vi "ManageRefs_FGV.vi"(7 "ManRef_mods":T1, 8 "error in":errorcluster, 11 "DataIn":variant) -> (0 "error out":errorcluster)   [LabVIEW 2017]
uses:
  ManRef_mods.ctl
  ManRef_data.ctl
  Asteroid_data.ctl
  GameConfig/GameConfig_data.ctl
  Asteroid_states.ctl
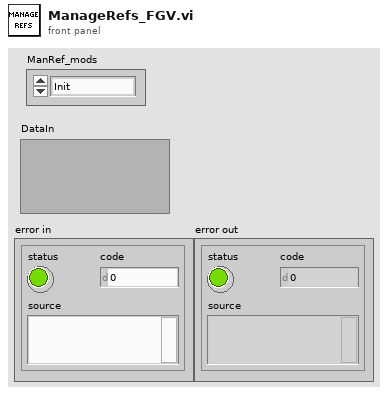
[diagram p1: front panel]
types:
  T1 = typedef "ManRef_mods.ctl" = enum16{"Init", "AddRef", "MoveAll", "DestroyRef", "End"}
  T2 = typedef "ManRef_data.ctl" = cluster{"ID":i32, "AsterObjectRef":refnum<vi>}
  T3 = typedef "Asteroid_states.ctl" = enum16{"Init", "Move", "Split", "Draw", "Destroy"}
  T4 = typedef "Asteroid_data.ctl" = cluster{"Veloc":dbl, "Direction":dbl, "Size":i32, "displayRef":refnum<vi>, "Max X":dbl, "Max Y":dbl, "Xpos":dbl, "Ypos":dbl, "ID":i32, "Config":T5}
  T5 = typedef "GameConfig_data.ctl" = cluster{"SpaceShip":cluster{"Angle":dbl, "SideLenght":dbl, "MaxLinearVeloc":dbl, "MaxAngularVeloc":dbl, "LinearAceleration":dbl, "AngularAceleration":dbl}, "Physics":cluster{"LinearDragFactor":dbl, "AngularDragFactor":dbl}, "Asteroids":cluster{"MaxSize":dbl, "MaxDivisions":i32, "MaxVeloc":dbl, "MinVeloc":dbl, "Fill":bool}, "Environment":cluster{"MaxAsteroids":i32, "TimeIncrement":dbl, "AsterProbCreation":dbl}}
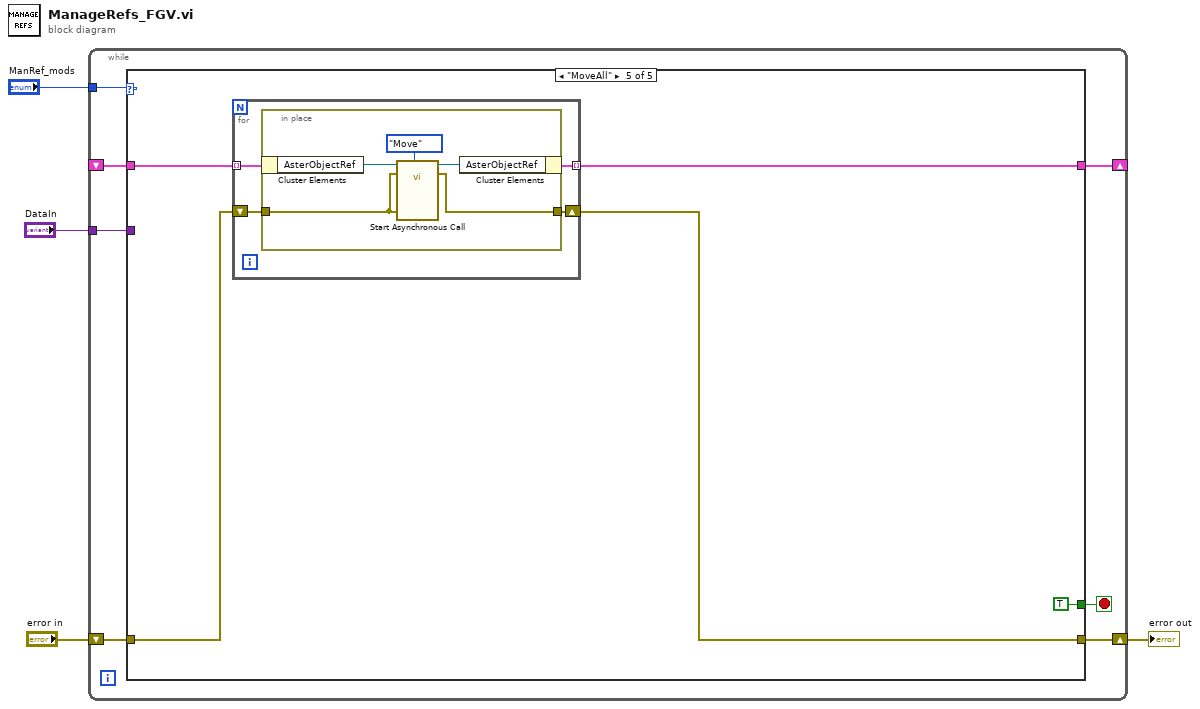
[diagram p0: block diagram]
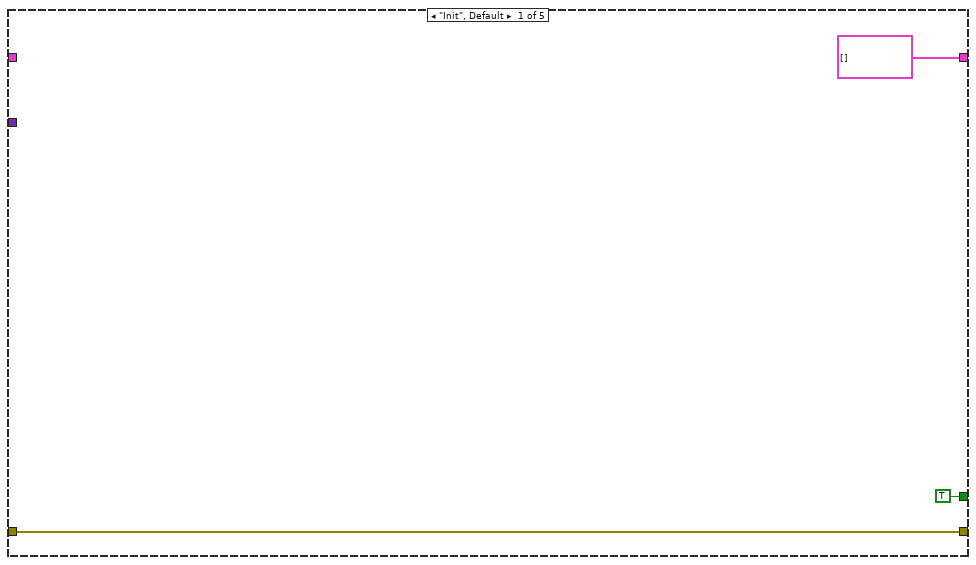
[diagram p2: hidden frame]
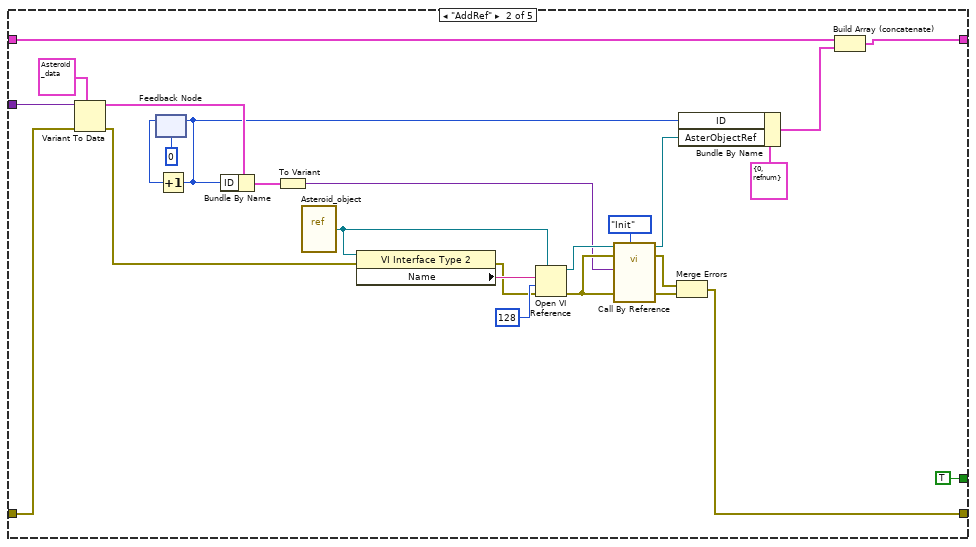
[diagram p3: hidden frame]
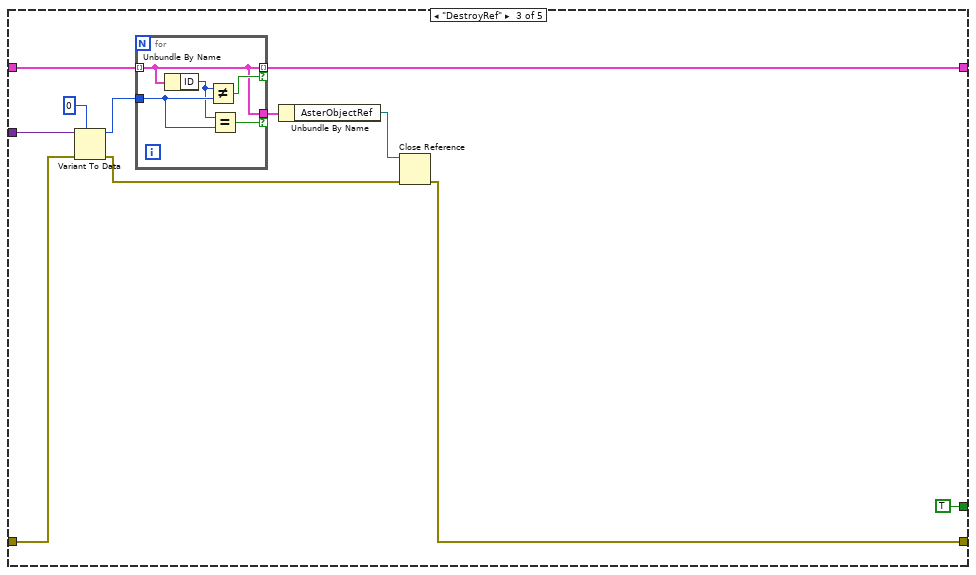
[diagram p4: hidden frame]
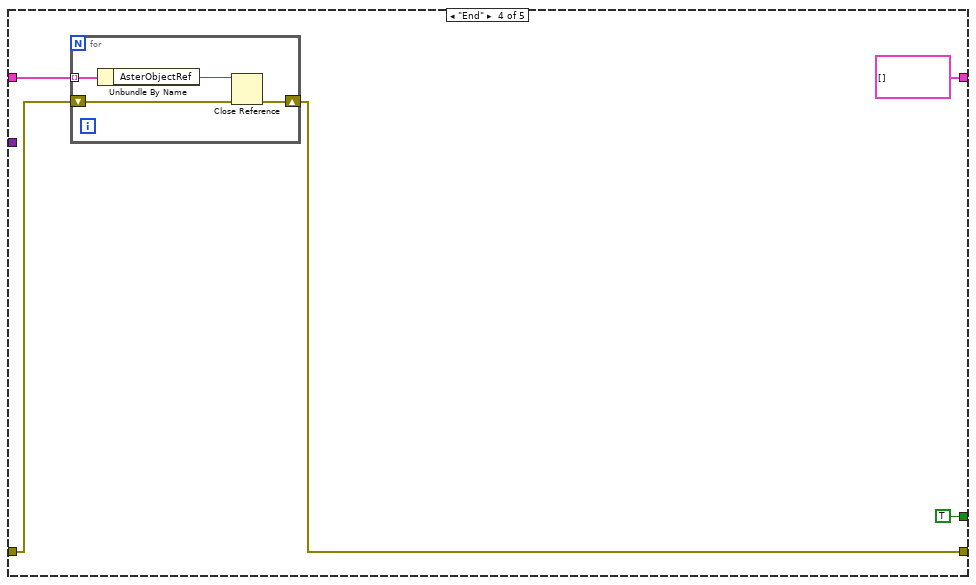
[diagram p5: hidden frame]
diagram:
  n1 = while {
    shift-right: [w8] -> w3
    shift-left: "error in" -> [w11]
    tunnel: "DataIn" -> [w10]
    tunnel: "ManRef_mods" -> [w9]
    shift-right: [w7] -> _
    shift-left: _ -> [w6]
    stop <- w5 stop-if-true
    n2 = case shown="\"MoveAll\"" w9 {
      tunnel: w11 -> [w14 w33 w50 w59 w69]
      tunnel: w10 -> [_ w35 w51 _ _]
      tunnel: [w14 w21 w41 w58 w67] -> w8
      tunnel: [T2[] [] ("appended array") w18 w46 T2[] [] ("appended array") w68] -> w7
      tunnel: w6 -> [_ w19 w47 w60 w70]
      tunnel: [TRUE ("empty?") TRUE ("empty?") TRUE ("empty?") TRUE ("empty?") TRUE ("empty?")] -> w5
      frame "Init", Default {
      }
      frame "AddRef" {
        n3 = Variant To Data(error in=w33, type=T4 {"Veloc"=0.0, "Direction"=0.0, "Size"=0, "displayRef"=refnum, "Max X"=0.0, "Max Y"=0.0, "Xpos"=0.0, "Ypos"=0.0, "ID"=0, "Config"={"SpaceShip"={"Angle"=30.0, "SideLenght"=2.0, "MaxLinearVeloc"=10.0, "MaxAngularVeloc"=10.0, "LinearAceleration"=1.0, "AngularAceleration"=1.0}, "Physics"={"LinearDragFactor"=1.0, "AngularDragFactor"=1.0}, "Asteroids"={"MaxSize"=6.0, "MaxDivisions"=3, "MaxVeloc"=8.0, "MinVeloc"=1.0, "Fill"=FALSE}, "Environment"={"MaxAsteroids"=10, "TimeIncrement"=0.1, "AsterProbCreation"=0.1}}} ("AsteroidData"), Variant=w35) -> (data=w26:T4, error out=w31:errorcluster)
        n4 = feedback #1(0) -> (w37:i32)
        n5 = Increment(x=w37) -> (x+1=w22:i32)
        n6 = feedback-in #1(w22) -> ()
        n7 = Bundle By Name(cluster=w26, "ID"=w22) -> (w25:T4)
        n8 = To Variant(anything=w25) -> (Variant=w24:variant)
        n9 = vi-ref "Asteroid_object.vi"() -> (w39:refnum<vi>)
        n10 = property class="VI Interface Type 2"(reference=w39, error in=w31) -> (error out=w30:errorcluster, "Name"=w40:string)  [unwired: 1 out]
        n11 = Open VI Reference(type specifier VI Refnum (for type only)=w39, vi path=w40, options=128, error in (no error)=w30) -> (vi reference=w34:refnum<vi>, error out=w29:errorcluster)  [unwired: 2 in]
        n12 = call-by-ref "?"(reference=w34, error in=w29, "Asteroid_states"=Asteroid_states."Init", "error in"=w29, "DataIn"=w24) -> (reference out=w16:refnum<vi>, error out=w27:errorcluster, 0:"error out"=w28:errorcluster)  [unwired: 7 in, 1 out]
        n13 = Merge Errors(w27, w28) -> (w21:errorcluster)
        n14 = Bundle By Name(cluster=T2 {"ID"=0, "AsterObjectRef"=refnum} ("DataCluster"), "ID"=w22, "AsterObjectRef"=w16) -> (w20:T2)
        n15 = Build Array (concatenate)(w19, w20) -> (w18:T2[])
      }
      frame "DestroyRef" {
        n16 = Variant To Data(error in=w50, type=0, Variant=w51) -> (data=w48:i32, error out=w42:errorcluster)
        n17 = for {
          tunnel: w47 -> [w53] mode=indexing
          tunnel: w48 -> [w55]
          tunnel: [w53] -> w46 mode=indexing if=w56
          tunnel: [w53] -> w45 if=w52
          n18 = Unbundle By Name(w53) -> ("ID"=w54:i32)
          n19 = Not Equal?(x=w54, y=w55) -> (x != y?=w56:bool)
          n20 = Equal?(x=w54, y=w55) -> (x = y?=w52:bool)
        }
        n21 = Unbundle By Name(w45) -> ("AsterObjectRef"=w43:refnum<vi>)
        n22 = Close Reference(reference=w43, error in (no error)=w42) -> (error out=w41:errorcluster)
      }
      frame "End" {
        n23 = for {
          tunnel: w60 -> [w65] mode=indexing
          shift-right: [w62] -> w58
          shift-left: w59 -> [w63]
          n24 = Unbundle By Name(w65) -> ("AsterObjectRef"=w64:refnum<vi>)
          n25 = Close Reference(reference=w64, error in (no error)=w63) -> (error out=w62:errorcluster)
        }
      }
      frame "MoveAll" {
        n26 = for {
          tunnel: w70 -> [w74] mode=indexing
          shift-right: [w72] -> w67
          shift-left: w69 -> [w73]
          tunnel: [w71] -> w68 mode=indexing
          n27 = in-place {
            in-place-border: w73 -> [w78]
            in-place-border: [w75] -> w72
            n28 = in-place-cluster #2(w74) -> ("AsterObjectRef"=w79:refnum<vi>)
            n29 = call-by-ref "Start Asynchronous Call"(reference=w79, error in=w78, "Asteroid_states"=Asteroid_states."Move", "error in"=w78) -> (reference out=w77:refnum<vi>, error out=w75:errorcluster)  [unwired: 8 in, 2 out]
            n30 = in-place-cluster #2("AsterObjectRef"=w77) -> (w71:T2)
          }
        }
      }
    }
  }
  "error out" <- w3
